vi "Fire-Sequence.vi"(0 "La Fire at will?":bool, 1 "Ready?":bool) -> (2 "Transfer":dbl, 3 "Fire!":bool, 4 "Set?":bool, 5 "Ready?":bool)   [LabVIEW 2012]
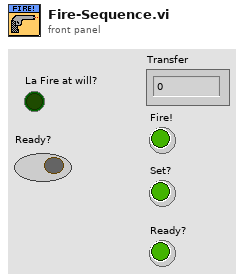
[diagram p1: front panel]
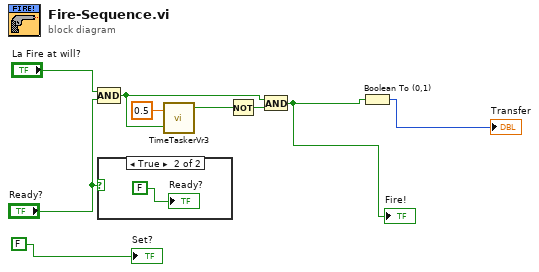
[diagram p0: block diagram]
diagram:
  n1 = Compound Arithmetic op=AND("La Fire at will?", "Ready?") -> (w6:bool)
  n2 = case shown="True" "Ready?" {
    frame False {
    }
    frame True {
      "Ready?" <- FALSE ("Set?")
    }
  }
  n3 = call "TimeTaskerVr3.vi"("Delay(sec)"=0.5, "Start Counting?"=w6) -> ("TimePast?"=w8:bool)  [unwired: 2 out]
  n4 = Not(x=w8) -> (.not. x?=w7:bool)
  n5 = And(x=w6, y=w7) -> (x .and. y?=w3:bool)
  "Fire!" <- w3
  n6 = Boolean To (0,1)(Boolean=w3) -> (0, 1=→"Transfer":i16)
  "Set?" <- FALSE ("Set?")
